vi "svx_SC Line Boundary.vi"(5 "start point":enum16{"center", "top", "bottom"}(ring), 6 "Boundary Color":u32(colorbox), 7 "boundary":cluster{"x axis":dbl, "y axis":dbl}, 10 "Shaft Centerline":refnum<vi>, 11 "Picture in":picture) -> (3 "Picture out":picture)   [LabVIEW 2017, in "SVX SC Line.xctl"]
uses:
  <vilib>/addons/_XControls/Shaft Centerline/SVX SC Line.xctl
panel:
  out "Shaft Centerline out":refnum<vi>
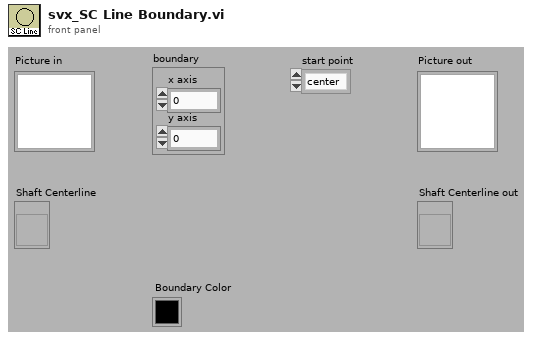
[diagram p1: front panel]
types:
  T1 = cluster{"Width":u16, "Style":enum32{"Solid", "Dash", "Dot", "DashDot", "DashDotDot"}}
  T2 = cluster{"left":i16, "top":i16, "right":i16, "bottom":i16}
  T3 = typedef "LVBoundsTypeDef.ctl" = cluster{"Width":u32, "Height":u32}
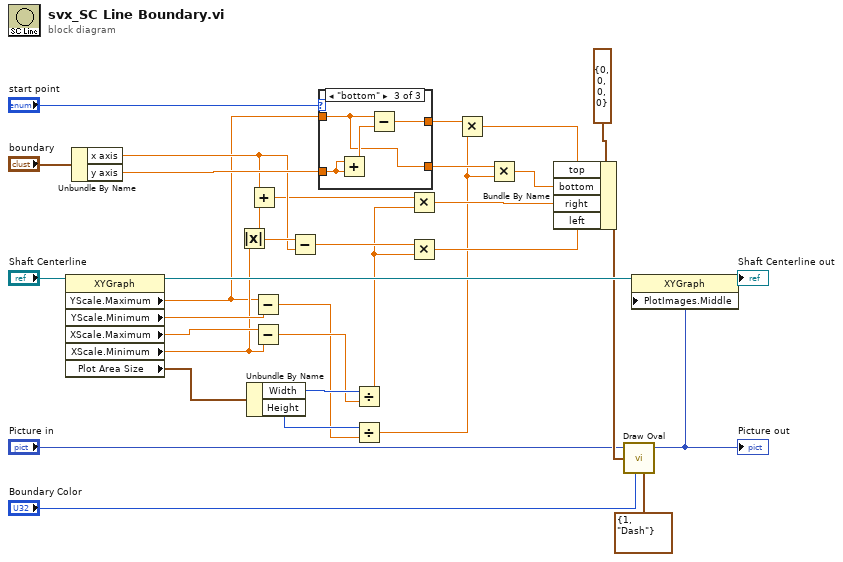
[diagram p0: block diagram]
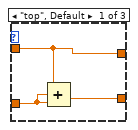
[diagram p2: hidden frame]
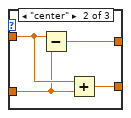
[diagram p3: hidden frame]
diagram:
  n1 = property class="XYGraph"(reference="Shaft Centerline") -> (reference out=w24:refnum<vi>, "YScale.Maximum"=w11:dbl, "YScale.Minimum"=w32:dbl, "XScale.Maximum"=w31:dbl, "XScale.Minimum"=w19:dbl, "Plot Area Size"=w30:T3)  [unwired: 1 in, 1 out]
  n2 = Unbundle By Name("boundary") -> ("x axis"=w17:dbl, "y axis"=w21:dbl)
  n3 = Absolute Value(x=w19) -> (abs(x)=w18:dbl)
  n4 = Unbundle By Name(w30) -> ("Width"=w29:u32, "Height"=w27:u32)
  n5 = Add(x=w17, y=w18) -> (x+y=w16:dbl)
  n6 = Subtract(x=w11, y=w32) -> (x-y=w26:dbl)
  n7 = Subtract(x=w31, y=w19) -> (x-y=w28:dbl)
  n8 = Subtract(x=w18, y=w17) -> (x-y=w15:dbl)
  n9 = case shown="\"bottom\"" "start point" {
    tunnel: w21 -> [w35 w38 w43]
    tunnel: w11 -> [w34 w39 w41]
    tunnel: [w34 w40 w44] -> w10
    tunnel: [w36 w37 w41] -> w9
    frame "top", Default {
      n10 = Compound Arithmetic op=ADD(w34, w35, w35) -> (w36:dbl)
    }
    frame "center" {
      n11 = Subtract(x=w39, y=w38) -> (x-y=w40:dbl)
      n12 = Add(x=w39, y=w38) -> (x+y=w37:dbl)
    }
    frame "bottom" {
      n13 = Add(x=w43, y=w43) -> (x+y=w42:dbl)
      n14 = Subtract(x=w41, y=w42) -> (x-y=w44:dbl)
    }
  }
  n15 = Divide(x=w29, y=w28) -> (x/y=w14:dbl)
  n16 = Divide(x=w27, y=w26) -> (x/y=w8:dbl)
  n17 = Multiply(x=w16, y=w14) -> (x*y=w12:dbl)
  n18 = Multiply(x=w15, y=w14) -> (x*y=w13:dbl)
  n19 = Multiply(x=w10, y=w8) -> (x*y=w7:dbl)
  n20 = Multiply(x=w9, y=w8) -> (x*y=w6:dbl)
  n21 = Bundle By Name(cluster=T2 {"left"=0, "top"=0, "right"=0, "bottom"=0} ("rect"), "top"=w7, "bottom"=w6, "right"=w12, "left"=w13) -> (w5:T2)
  n22 = call <vilib>:"Draw Oval.vi"("picture"="Picture in", "rect"=w5, "color(black)"="Boundary Color", "pen"=T1 {"Width"=1, "Style"=enum."Dash"}) -> ("new picture"=w1:picture)  [unwired: 5 in]
  "Picture out" <- w1
  n23 = property class="XYGraph"(reference=w24, "PlotImages.Middle"=w1) -> (reference out=→"Shaft Centerline out":refnum<vi>)  [unwired: 1 in, 1 out]
